vi "PRL BUFFER Rearrange Analog 2D Array.vi"(10 "Cut Index":i32, 11 "Array In":sgl[][](array[numeric])) -> (3 "Array Out":sgl[][](array[numeric]))   [LabVIEW 2018, in "S3DK.lvlib" / "PMU Recorder Light.lvlib"]
uses:
  PMU Recorder Light.lvlib
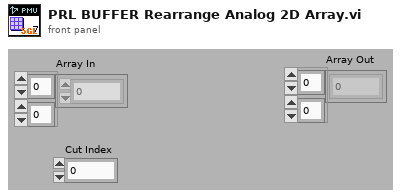
[diagram p1: front panel]
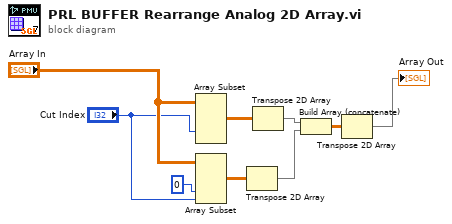
[diagram p0: block diagram]
diagram:
  n1 = Array Subset(array="Array In", index (col)="Cut Index") -> (w9:sgl[][])  [unwired: 3 in]
  n2 = Array Subset(array="Array In", index (col)=0 ("index"), length (col)="Cut Index") -> (w8:sgl[][])  [unwired: 2 in]
  n3 = Transpose 2D Array(2D array=w8) -> (transposed array=w2:sgl[][])
  n4 = Transpose 2D Array(2D array=w9) -> (transposed array=w3:sgl[][])
  n5 = Build Array (concatenate)(w3, w2) -> (w6:sgl[][])
  n6 = Transpose 2D Array(2D array=w6) -> (transposed array=→"Array Out":sgl[][])
